vi "(Depricated) Handle Timeout Syringe.vi"(8 "error in (no error)":errorcluster, 9 "Syringe Pressure Raw":dbl, 10 "Syringe Pressure mean":dbl, 11 "cRIO Vacuum in":refnum<class "cRIO Vacuum.lvclass">) -> (0 "error out":errorcluster, 3 "cRIO Vacuum out":refnum<class "cRIO Vacuum.lvclass">)   [LabVIEW 2015]
uses:
  Controls/Vacuum State Enumerator.ctl
  cRIO Vacuum.lvclass
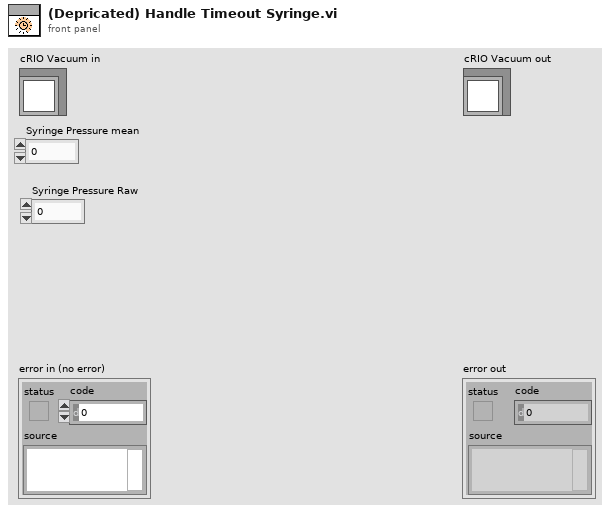
[diagram p1: front panel]
types:
  T1 = typedef "Vacuum State Enumerator.ctl" = enum16{"Pressure Rising", "Plateau", "Pressure Dropping", "Valley", "Low Valley", "Leak", "Unknown"}
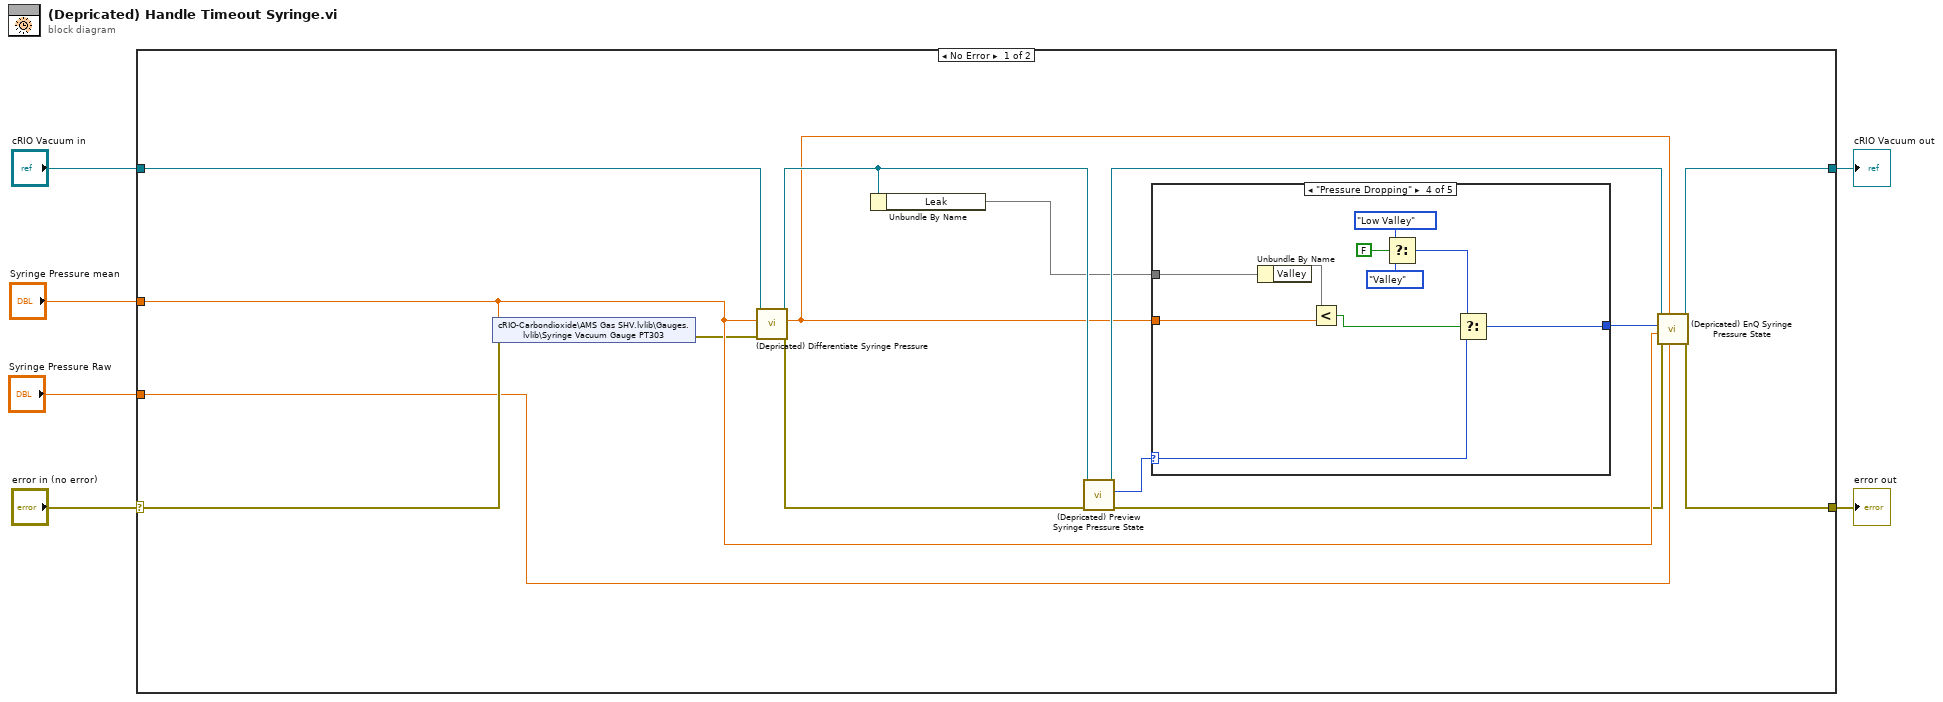
[diagram p0: block diagram]
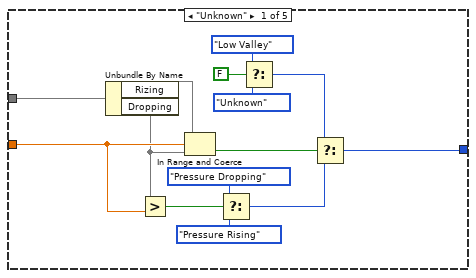
[diagram p2: hidden frame]
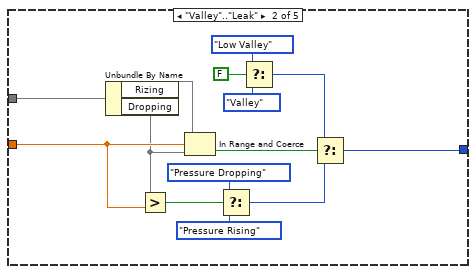
[diagram p3: hidden frame]
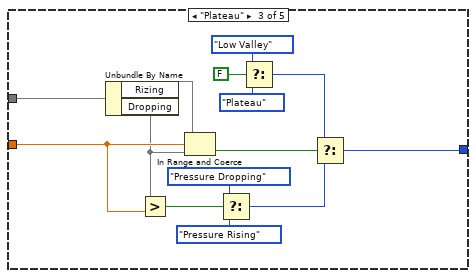
[diagram p4: hidden frame]
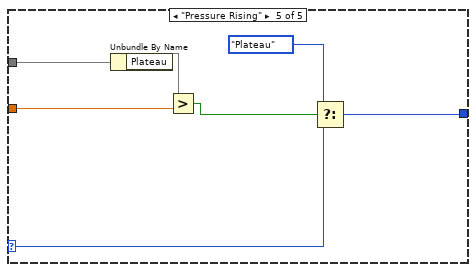
[diagram p5: hidden frame]
diagram:
  n1 = case shown="No Error" "error in (no error)" {
    selector: "error in (no error)" -> [w9 w82]
    tunnel: [w19 w82] -> w5
    tunnel: [w20 w81] -> w3
    tunnel: "cRIO Vacuum in" -> [w21 w81]
    tunnel: "Syringe Pressure mean" -> [w18 _]
    tunnel: "Syringe Pressure Raw" -> [w7 _]
    frame No Error {
      n2 = shared-variable "cRIO-Carbondioxide\\AMS Gas SHV.lvlib\\Gauges.lvlib\\Syringe Vacuum Gauge PT303"(w18, error in=w9) -> (error out=w8:errorcluster)
      n3 = call "(Depricated) Differentiate Syringe Pressure.vi"("error in (no error)"=w8, "Syringe Pressure"=w18, "cRIO Vacuum in"=w21) -> ("error out"=w12:errorcluster, "d/dt"=w10:dbl, "cRIO Vacuum out"=w13:refnum<class "cRIO Vacuum.lvclass">)  [unwired: 6 in]
      n4 = Unbundle By Name(w13) -> ("Leak"=w11)
      n5 = call "(Depricated) Preview Syringe Pressure State.vi"("error in (no error)"=w12, "cRIO Vacuum in"=w13) -> ("error out"=w16:errorcluster, "Syringe Pressure State"=w17:T1, "cRIO Vacuum out"=w14:refnum<class "cRIO Vacuum.lvclass">)  [unwired: 3 in, 4 out]
      n6 = case shown="\"Pressure Dropping\"" w17 {
        selector: w17 -> [_ _ _ w65 w75]
        tunnel: w11 -> [w35 w49 w63 w73 w80]
        tunnel: w10 -> [w31 w46 w59 w67 w77]
        tunnel: [w23 w36 w51 w69 w79] -> w15
        frame "Unknown" {
          n7 = Unbundle By Name(w35) -> ("Rizing"=w34, "Dropping"=w30)
          n8 = Greater?(x=w30, y=w31) -> (0:w32:bool)
          n9 = In Range and Coerce(upper limit=w34, x=w31, lower limit=w30) -> (In Range?=w33:bool)  [unwired: 1 out]
          n10 = Select(t=Vacuum_State_Enumerator."Pressure Dropping" ("Vacuum State"), s=w32, f=Vacuum_State_Enumerator."Pressure Rising") -> (s? t:f=w29:T1)
          n11 = Select(t=Vacuum_State_Enumerator."Low Valley", s=FALSE, f=Vacuum_State_Enumerator."Unknown" ("Vacuum State")) -> (s? t:f=w24:T1)
          n12 = Select(t=w24, s=w33, f=w29) -> (s? t:f=w23:T1)
        }
        frame "Valley".."Leak" {
          n13 = Unbundle By Name(w49) -> ("Rizing"=w48, "Dropping"=w45)
          n14 = Greater?(x=w45, y=w46) -> (0:w47:bool)
          n15 = In Range and Coerce(upper limit=w48, x=w46, lower limit=w45) -> (In Range?=w38:bool)  [unwired: 1 out]
          n16 = Select(t=Vacuum_State_Enumerator."Pressure Dropping" ("Vacuum State"), s=w47, f=Vacuum_State_Enumerator."Pressure Rising") -> (s? t:f=w44:T1)
          n17 = Select(t=Vacuum_State_Enumerator."Low Valley", s=FALSE, f=Vacuum_State_Enumerator."Valley" ("Vacuum State")) -> (s? t:f=w39:T1)
          n18 = Select(t=w39, s=w38, f=w44) -> (s? t:f=w36:T1)
        }
        frame "Plateau" {
          n19 = Unbundle By Name(w63) -> ("Rizing"=w62, "Dropping"=w58)
          n20 = Greater?(x=w58, y=w59) -> (0:w60:bool)
          n21 = In Range and Coerce(upper limit=w62, x=w59, lower limit=w58) -> (In Range?=w61:bool)  [unwired: 1 out]
          n22 = Select(t=Vacuum_State_Enumerator."Pressure Dropping" ("Vacuum State"), s=w60, f=Vacuum_State_Enumerator."Pressure Rising") -> (s? t:f=w57:T1)
          n23 = Select(t=Vacuum_State_Enumerator."Low Valley", s=FALSE, f=Vacuum_State_Enumerator."Plateau" ("Vacuum State")) -> (s? t:f=w52:T1)
          n24 = Select(t=w52, s=w61, f=w57) -> (s? t:f=w51:T1)
        }
        frame "Pressure Dropping" {
          n25 = Unbundle By Name(w73) -> ("Valley"=w68)
          n26 = Less?(x=w68, y=w67) -> (x < y?=w66:bool)
          n27 = Select(t=Vacuum_State_Enumerator."Low Valley", s=FALSE, f=Vacuum_State_Enumerator."Valley" ("Vacuum State")) -> (s? t:f=w70:T1)
          n28 = Select(t=w70, s=w66, f=w65) -> (s? t:f=w69:T1)
        }
        frame "Pressure Rising" {
          n29 = Unbundle By Name(w80) -> ("Plateau"=w78)
          n30 = Greater?(x=w78, y=w77) -> (0:w76:bool)
          n31 = Select(t=Vacuum_State_Enumerator."Plateau", s=w76, f=w75) -> (s? t:f=w79:T1)
        }
      }
      n32 = call "(Depricated) EnQ Syringe Pressure State.vi"("Raw Pressure"=w7, "d/dt"=w10, "error in (no error)"=w16, "Pressure"=w18, "State"=w15, "cRIO Vacuum in"=w14) -> ("error out"=w19:errorcluster, "cRIO Vacuum out"=w20:refnum<class "cRIO Vacuum.lvclass">)  [unwired: 4 out]
    }
    frame Error {
    }
  }
  "error out" <- w5
  "cRIO Vacuum out" <- w3
